vi "Set LED Mode.vi"(8 "error in":errorcluster {"code" format="%.0x"}, 10 "Mode":string, 11 "Session In":refnum<visa-resource-name>) -> (0 "error out":errorcluster {"code" format="%.0x"}, 3 "Session Out":refnum<visa-resource-name>)   [LabVIEW 2012, in "YOST 3 Space.lvlib"]
uses:
  YOST 3 Space.lvlib
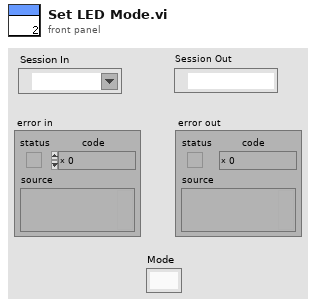
[diagram p1: front panel]
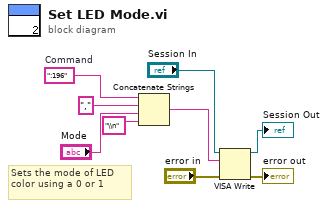
[diagram p0: block diagram]
diagram:
  w7 = ":196"  # Command
  # "Sets the mode of LED color using a 0 or 1"
  n1 = Concatenate Strings(w7, "," ("string"), "Mode", "\\n" ("string")) -> (w6:string)
  n2 = VISA Write(VISA resource name="Session In", write buffer=w6, error in (no error)="error in") -> (VISA resource name out=→"Session Out":refnum<visa-resource-name>, error out=→"error out":errorcluster)  [unwired: 1 out]
